vi "Polynomordnung.vi"(10 "LIN Polynom":dbl[](array[numeric]) format="%#_18f") -> (2 "LIN Polynom out":dbl[](array[numeric]) format="%#_18f", 3 "Polynomordnung":i32)   [LabVIEW 2020, in "Linearisierung v2.lvlib"]
uses:
  Linearisierung v2.lvlib
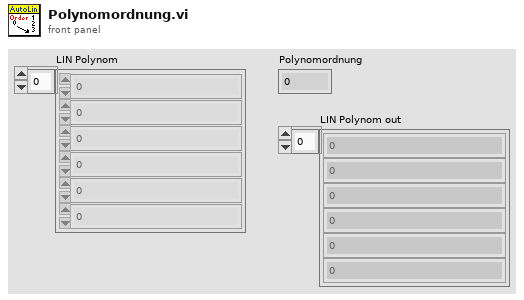
[diagram p1: front panel]
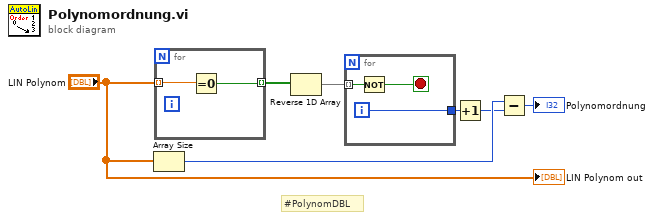
[diagram p0: block diagram]
diagram:
  # "#PolynomDBL"
  n1 = Array Size(array="LIN Polynom") -> (size(s)=w3:i32)
  n2 = for {
    tunnel: "LIN Polynom" -> [w9] mode=indexing
    tunnel: [w8] -> w7 mode=indexing
    n3 = Equal To 0?(x=w9) -> (x = 0?=w8:bool)
  }
  n4 = Reverse 1D Array(array=w7) -> (reversed array=w6:bool[])
  n5 = for {
    tunnel: w6 -> [w12] mode=indexing
    tunnel: [w10] -> w4
    i -> [w10]
    stop <- w11 stop-if-true
    n6 = Not(x=w12) -> (.not. x?=w11:bool)
  }
  n7 = Increment(x=w4) -> (x+1=w2:i32)
  n8 = Subtract(x=w3, y=w2) -> (x-y=→"Polynomordnung":i32)
  "LIN Polynom out" <- "LIN Polynom"
